vi "Stop Core.vi"(10 "final error code":i32, 11 "Iterator Actor in":refnum<class "Iterator NR Actor.lvclass">) -> (3 "Iterator Actor out":refnum<class "Iterator NR Actor.lvclass">)   [LabVIEW 2023, in "Iterator Actor.lvlib" / "Iterator NR Actor.lvclass"]
doc: "(<B>Filename</B>: Actor Framework.lvlib:Actor.lvclass:Stop Core.vi)\n\nDefines what the actor does before it stops. Use the <B>final error code</B> input to determine whether the actor shut down in response to an error.\n\nBy default, this method does nothing. A descendant class may override it to define behavior, such as shutting down any processes the actor initiated in its override of the Actor Core method."
uses:
  Iterator NR Actor.lvclass
  Iterator NR Actor.lvclass/Iterator NR Actor.ctl
  Abstract Iterator Actor/Abstract Iterator Actor.lvclass
  <userlib>/_OpenG.lib/error/error.llb/openg_error.lvlib
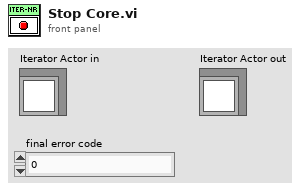
[diagram p1: front panel]
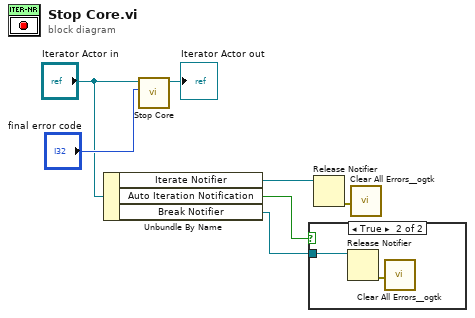
[diagram p0: block diagram]
diagram:
  n1 = Unbundle By Name("Iterator Actor in") -> ("Iterate Notifier"=w4:refnum<notifier>, "Auto Iteration Notification"=w2:bool, "Break Notifier"=w1:refnum<notifier>)
  n2 = call-parent "Stop Core.vi"("final error code"="final error code", "Iterator Actor in"="Iterator Actor in") -> ("Iterator Actor out"=→"Iterator Actor out":refnum<class "Iterator NR Actor.lvclass">)  [unwired: 9 in]
  n3 = case shown="True" w2 {
    tunnel: w1 -> [_ w8]
    frame False {
    }
    frame True {
      n4 = Release Notifier(notifier=w8) -> (error out=w9:errorcluster)  [unwired: 2 in, 2 out]
      n5 = call <userlib>:"Clear All Errors__ogtk.vi"("Error In"=w9) -> ()  [unwired: 3 in, 1 out]
    }
  }
  n6 = Release Notifier(notifier=w4) -> (error out=w3:errorcluster)  [unwired: 2 in, 2 out]
  n7 = call <userlib>:"Clear All Errors__ogtk.vi"("Error In"=w3) -> ()  [unwired: 3 in, 1 out]
